vi "Get command.vi"(8 "error in (no error)":errorcluster, 11 "Messenger in":refnum<class "Messenger.lvclass">) -> (0 "error out":errorcluster, 1 "isAcommand":bool, 2 "command":string, 3 "Messenger out":refnum<class "Messenger.lvclass">)   [LabVIEW 2018, in "Messenger.lvclass"]
uses:
  Messenger.lvclass
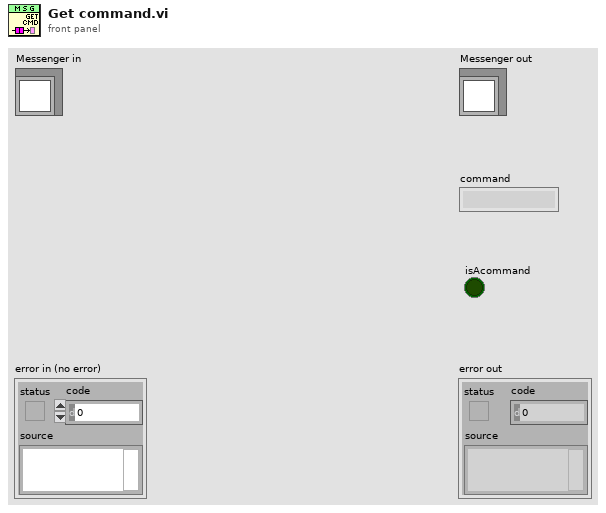
[diagram p1: front panel]
types:
  T1 = typedef "Message Queue.lvlib/Message Cluster.ctl" = cluster{"Message":string, "Message Data":variant}
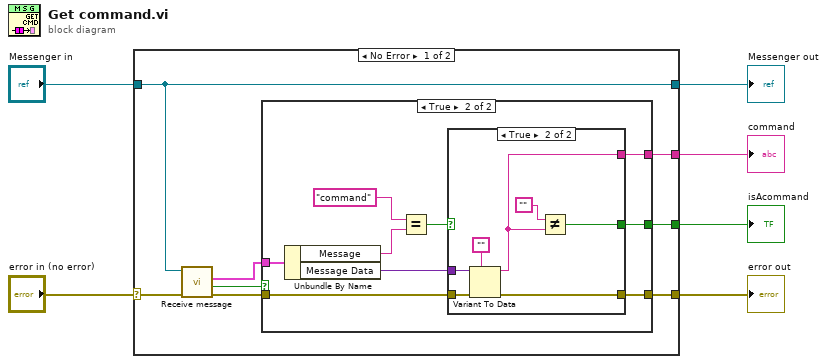
[diagram p0: block diagram]
diagram:
  n1 = case shown="No Error" "error in (no error)" {
    selector: "error in (no error)" -> [w14 w35]
    tunnel: [w9 w35] -> w5
    tunnel: [w7 w36] -> w3
    tunnel: "Messenger in" -> [w7 w36]
    tunnel: [w10 _] -> w2
    tunnel: [w8 _] -> w1
    frame No Error {
      n2 = call-dynamic "Receive message.vi"("error in (no error)"=w14, "Messenger in"=w7) -> ("error out"=w13:errorcluster, "new msg"=w12:bool, "message"=w11:T1)  [unwired: 6 in, 1 out]
      n3 = case shown="True" w12 {
        selector: w12 -> [w16 _]
        tunnel: w13 -> [w15 w22]
        tunnel: w11 -> [_ w21]
        tunnel: [w16 w20] -> w10
        tunnel: [w15 w19] -> w9
        tunnel: [_ w18] -> w8
        frame False {
        }
        frame True {
          n4 = Unbundle By Name(w21) -> ("Message"=w25:string, "Message Data"=w23:variant)
          n5 = Equal?(x="command", y=w25) -> (x = y?=w17:bool)
          n6 = case shown="True" w17 {
            selector: w17 -> [w26 _]
            tunnel: w23 -> [_ w34]
            tunnel: w22 -> [w27 w33]
            tunnel: [_ w29] -> w18
            tunnel: [w26 w28] -> w20
            tunnel: [w27 w31] -> w19
            frame False {
            }
            frame True {
              n7 = Variant To Data(error in=w33, type="", Variant=w34) -> (data=w29:string, error out=w31:errorcluster)
              n8 = Not Equal?(x="", y=w29) -> (x != y?=w28:bool)
            }
          }
        }
      }
    }
    frame Error {
    }
  }
  "error out" <- w5
  "Messenger out" <- w3
  "isAcommand" <- w2
  "command" <- w1
